vi "dodaj kursory pom.vi"(6 "Kolor":u32(colorbox)=16776704, 7 "Wektor przebiegow":waveform(dbl)[](array[waveform]), 8 "error in (no error)":errorcluster, 11 "Wykres Ref":refnum<vi>) -> (0 "error out":errorcluster)   [LabVIEW 2014]
doc: "Use this template to build a VI to use as a subVI."
uses:
  <vilib>/measure/NI_MABase.lvlib
panel:
  in  "Kursor 2":string="Kursor 2"
  in  "Przebieg 2":i32(ring) items=["Kana³ A", "Predkosc", "Przysp", "Kana³ 1, V", "Kana³ 2, V", "DI1"]
  in  "Przebieg 1":i32(ring) items=["Kana³ A", "Predkosc", "Przysp", "Kana³ 1, V", "Kana³ 2, V", "DI1"]
  in  "Array":T1(array[cluster])=[{"signal type"=enum."Sine Wave", "frequency"=10.0, "amplitude"=2.0}, {"signal type"=enum."Sine Wave", "frequency"=13.0, "amplitude"=1.0}, {"signal type"=enum."Sine Wave", "frequency"=7.0, "amplitude"=1.0}, {"signal type"=enum."Sine Wave", "frequency"=5.0, "amplitude"=3.0}] {"amplitude" format="%0.2p"; "frequency" format="%0.2p"}
  in  "Cancel":bool
  in  "OK":bool
  in  "Kursor 1":string="Kursor 1"
  # "UWAGA prosta ³¹cz¹ca punkty pomiarowe pojawia siê TYLKO wtedy,\nkiedy obydwa kursory pracuj¹ na przebiegach w tej samej skali"
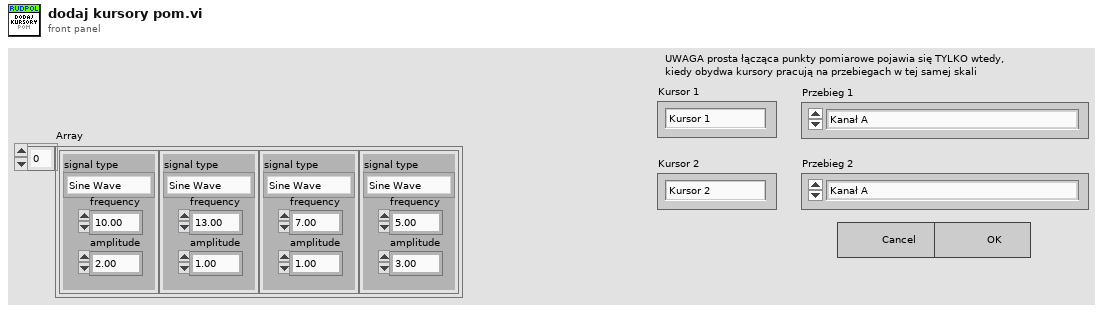
[diagram p1: front panel]
types:
  T1 = cluster{"signal type":enum16{"Sine Wave", "Triangle Wave", "Square Wave", "Sawtooth Wave"}, "frequency":dbl, "amplitude":dbl}[]
  T2 = enum16{"Sine Wave", "Triangle Wave", "Square Wave", "Sawtooth Wave"}
  T3 = typedef "LVCursorListTypeDef.ctl" = cluster{"Name":string, "Color":u32, "Style":u8, "Point Style":u8, "Name Visible":bool, "Allow Drag":bool, "Cursor Mode":u32, "Plot":i32, "Index":i32, "Position":cluster{"X":dbl, "Y":dbl}, "X Scale":u32, "Y Scale":u32, "Watch Plots":i32[], "Watch All Plots":bool, "Plot Area":i32, "Label Offset":cluster{"X":dbl, "Y":dbl}}[]
  T4 = cluster{"Name":string, "Color":u32, "Style":u8, "Point Style":u8, "Name Visible":bool, "Allow Drag":bool, "Cursor Mode":u32, "Plot":i32, "Index":i32, "Position":cluster{"X":dbl, "Y":dbl}, "X Scale":u32, "Y Scale":u32, "Watch Plots":i32[], "Watch All Plots":bool, "Plot Area":i32, "Label Offset":cluster{"X":dbl, "Y":dbl}}
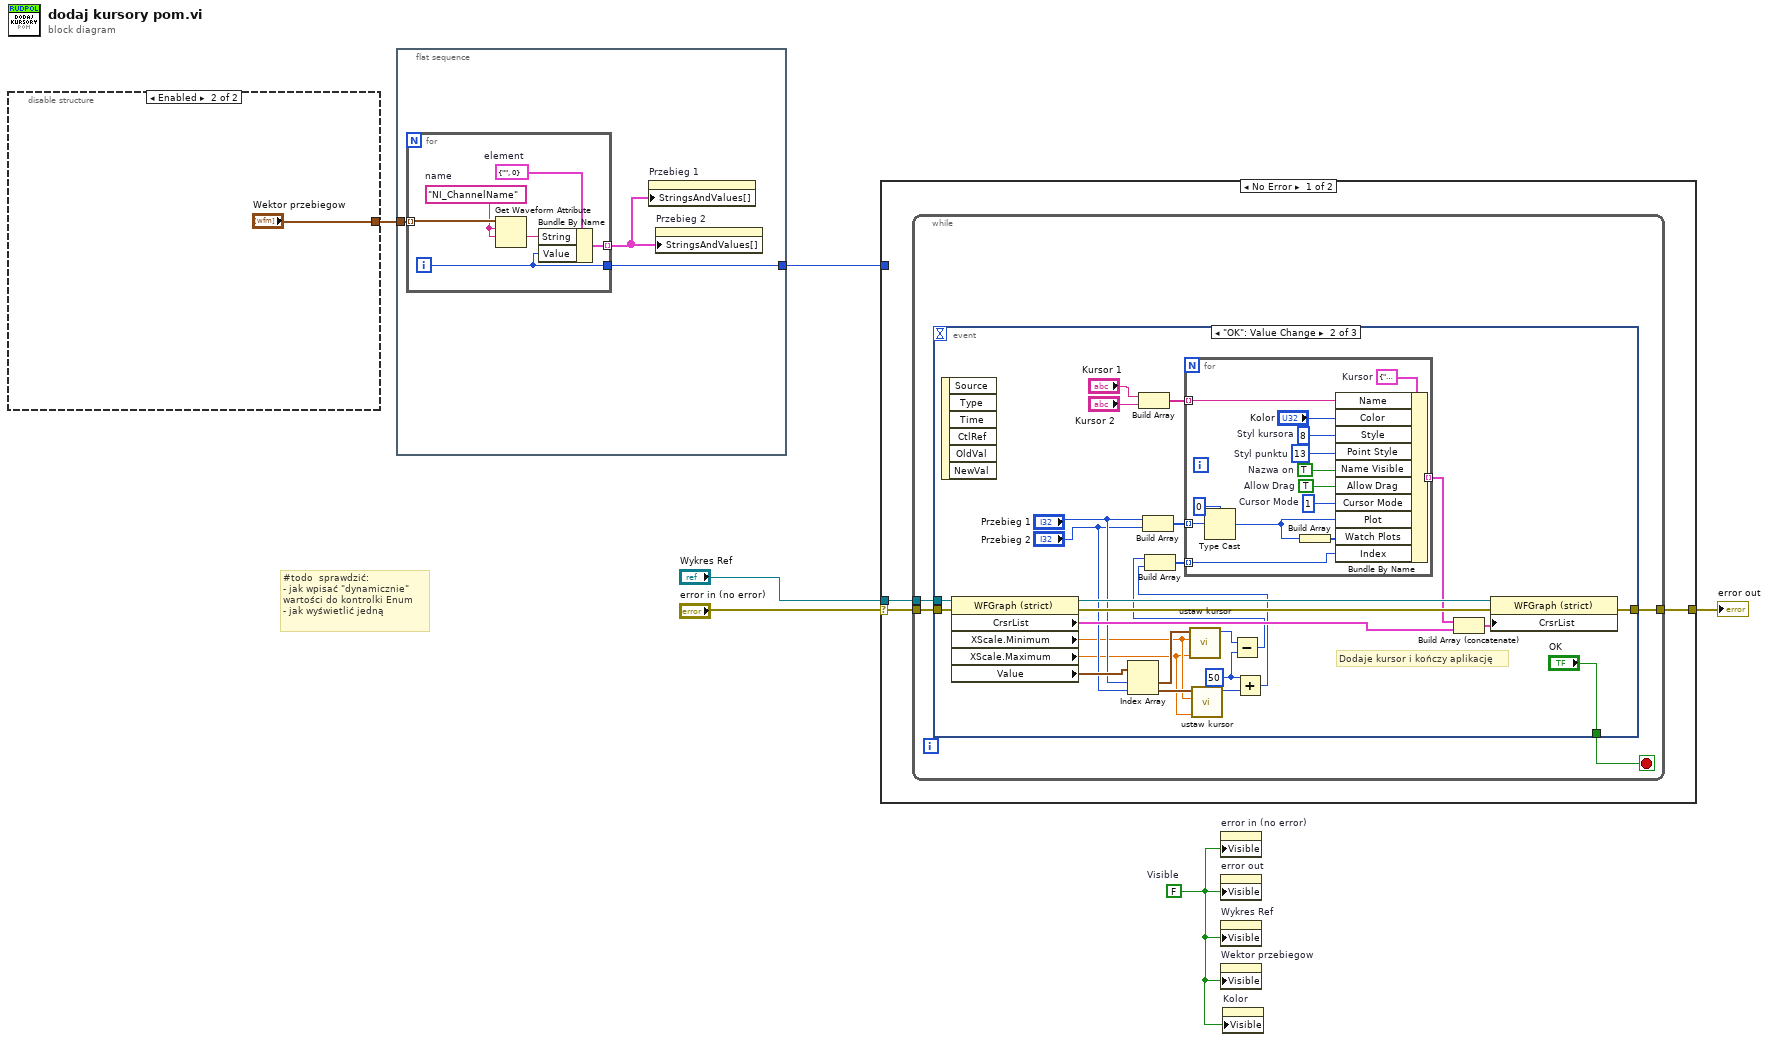
[diagram p0: block diagram]
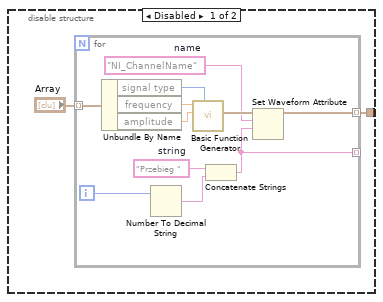
[diagram p2: hidden frame]
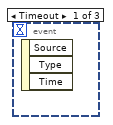
[diagram p3: hidden frame]
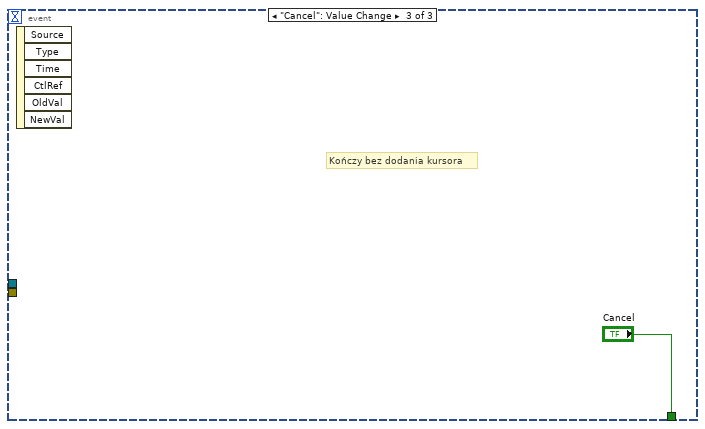
[diagram p4: hidden frame]
diagram:
  w1 = FALSE  # Visible
  # "#todo  sprawdziæ:\n- jak wpisaæ \"dynamicznie\"\nwartoœci do kontrolki Enum\n- jak wyœwietliæ jedn¹"
  n1 = disable-structure shown="Enabled" {
    disable-tunnel: [w7 "Wektor przebiegow"] -> w3
    frame Disabled {
      n2 = for {
        tunnel: "Array" -> [w16] mode=indexing
        tunnel: [w10] -> w7 mode=indexing
        tunnel: [w9] -> _ mode=indexing
        i -> [w11]
        w13 = "Przebieg "  # string
        w14 = "NI_ChannelName"  # name
        n3 = Unbundle By Name(w16) -> ("signal type"=w19:T2, "frequency"=w18:dbl, "amplitude"=w17:dbl)
        n4 = Number To Decimal String(number=w11) -> (decimal integer string=w12:string)  [unwired: 1 in]
        n5 = call <vilib>:"Basic Function Generator.vi"("signal type"=w19, "amplitude"=w17, "frequency"=w18) -> ("signal out"=w15:waveform(dbl))  [unwired: 6 in, 2 out]
        n6 = Concatenate Strings(w13, w12) -> (w9:string)
        n7 = Set Waveform Attribute(5:w9, 6:w14, 7:w15) -> (3:w10:waveform(dbl))  [unwired: 1 in, 2 out]
      }
    }
    frame Enabled {
    }
  }
  n8 = flat-sequence {
    tunnel: w3 -> [w23]
    tunnel: [w21] -> w2
    frame #0 {
      n9 = for {
        tunnel: w23 -> [w29] mode=indexing
        tunnel: [w25] -> w21
        tunnel: [w24] -> w22 mode=indexing
        i -> [w25]
        w27 = cluster{"String":string, "Value":u16} {"String"="", "Value"=0}  # element
        w28 = "NI_ChannelName"  # name
        n10 = Get Waveform Attribute(5:w28, 6:w28, 7:w29) -> (1:w26:string)  [unwired: 1 in, 3 out]
        n11 = Bundle By Name(cluster=w27, "String"=w26, "Value"=w25) -> (w24:cluster{"String":string, "Value":u16})
      }
      n12 = property on="Przebieg 1" class="Ring (strict)"("StringsAndValues[]"=w22) -> ()  [unwired: 2 in, 2 out]
      n13 = property on="Przebieg 2" class="Ring (strict)"("StringsAndValues[]"=w22) -> ()  [unwired: 2 in, 2 out]
    }
  }
  n14 = case shown="No Error" "error in (no error)" {
    selector: "error in (no error)" -> [w32 w78]
    tunnel: [w31 w78] -> w5
    tunnel: "Wykres Ref" -> [w30 _]
    tunnel: w2 -> [_ _]
    frame No Error {
      n15 = while {
        tunnel: w32 -> [w34]
        tunnel: [w33] -> w31
        tunnel: w30 -> [w36]
        stop <- w35 stop-if-true
        n16 = event shown="[1] \"OK\": Value Change" {
          selector: _ -> [_ _ _]
          dyn-events: _ -> [_ _ _]
          timeout: _ -> [_ _ _]
          tunnel: w36 -> [_ w61 _]
          tunnel: [_ "OK" "Cancel"] -> w35
          tunnel: w34 -> [_ w60 _]
          tunnel: [_ w57 _] -> w33
          event Timeout {
            n17 = event-data() -> ()  [unwired: 1 in, 3 out]
          }
          event "OK": Value Change {
            w39 = 50 ("x")
            # "Dodaje kursor i koñczy aplikacjê"
            n18 = event-data() -> ()  [unwired: 1 in, 6 out]
            n19 = property class="WFGraph (strict)"(reference=w61, error in=w60) -> (reference out=w59:refnum<vi>, error out=w58:errorcluster, "CrsrList"=w54:T3, "XScale.Minimum"=w43:dbl, "XScale.Maximum"=w42:dbl, "Value"=w48:waveform(dbl)[])
            n20 = Index Array(array=w48, index #1="Przebieg 1", index #2="Przebieg 2") -> (element #1=w45:waveform(dbl), element #2=w44:waveform(dbl))
            n21 = Build Array("Kursor 1", "Kursor 2") -> (w49:string[])
            n22 = Build Array("Przebieg 1", "Przebieg 2") -> (w52:i32[])
            n23 = call "ustaw kursor.vi"("XScale.Maximum"=w42, "XScale.Minimum"=w43, "signal in"=w45) -> ("Index"=w41:i32)  [unwired: 6 in, 2 out]
            n24 = call "ustaw kursor.vi"("XScale.Maximum"=w42, "XScale.Minimum"=w43, "signal in"=w44) -> ("Index"=w40:i32)  [unwired: 6 in, 2 out]
            n25 = Subtract(x=w41, y=w39) -> (x-y=w37:i32)
            n26 = Add(x=w39, y=w40) -> (x+y=w38:i32)
            n27 = Build Array(w37, w38) -> (w51:i32[])
            n28 = for {
              tunnel: [w66] -> w55 mode=indexing
              tunnel: w52 -> [w65] mode=indexing
              tunnel: w51 -> [w64] mode=indexing
              tunnel: w49 -> [w63] mode=indexing
              w73 = u8 13  # Styl punktu
              w74 = u8 8  # Styl kursora
              w72 = TRUE  # Nazwa on
              w67 = u32 1  # Cursor Mode
              w71 = TRUE  # Allow Drag
              w76 = T4 {"Name"="", "Color"=0, "Style"=0, "Point Style"=0, "Name Visible"=FALSE, "Allow Drag"=FALSE, "Cursor Mode"=0, "Plot"=0, "Index"=0, "Position"={"X"=0.0, "Y"=0.0}, "X Scale"=0, "Y Scale"=0, "Watch Plots"=[], "Watch All Plots"=FALSE, "Plot Area"=0, "Label Offset"={"X"=0.0, "Y"=0.0}}  # Kursor
              n29 = Type Cast(type=0, x=w65) -> (*(type *) &x=w68:i32)
              n30 = Build Array(w68) -> (w69:i32[])
              n31 = Bundle By Name(cluster=w76, "Name"=w63, "Color"="Kolor", "Style"=w74, "Point Style"=w73, "Name Visible"=w72, "Allow Drag"=w71, "Cursor Mode"=w67, "Plot"=w68, "Watch Plots"=w69, "Index"=w64) -> (w66:T4)
            }
            n32 = Build Array (concatenate)(w55, w54) -> (w56:T3)
            n33 = property class="WFGraph (strict)"(reference=w59, error in=w58, "CrsrList"=w56) -> (error out=w57:errorcluster)  [unwired: 1 out]
          }
          event "Cancel": Value Change {
            # "Koñczy bez dodania kursora"
            n34 = event-data() -> ()  [unwired: 1 in, 6 out]
          }
        }
      }
    }
    frame Error {
    }
  }
  "error out" <- w5
  n35 = property on="error in (no error)" class="Clust (strict)"("Visible"=w1) -> ()  [unwired: 2 in, 2 out]
  n36 = property on="error out" class="Clust (strict)"("Visible"=w1) -> ()  [unwired: 2 in, 2 out]
  n37 = property on="Wykres Ref" class="LVObjRef (strict)"("Visible"=w1) -> ()  [unwired: 2 in, 2 out]
  n38 = property on="Wektor przebiegow" class="Arr (strict)"("Visible"=w1) -> ()  [unwired: 2 in, 2 out]
  n39 = property on="Kolor" class="ColBox"("Visible"=w1) -> ()  [unwired: 2 in, 2 out]
